vi "Find Timeout.vi"(0 "State in":refnum<class "State.lvclass">, 7 "Type":T1, 11 "error in (no error)":errorcluster) -> (4 "State thru":refnum<class "State.lvclass">, 8 "Timeout":refnum<class "Timeout.lvclass">, 15 "error out":errorcluster)   [LabVIEW 2020, in "State.lvclass"]
uses:
  State.lvclass
  Typedefs/Tosca-Event Type.ctl
  Timeout/Timeout.lvclass
  State.lvclass/State.ctl
  Timeout/Timeout.lvclass/Timeout.ctl
  Timeout/Read Type.vi
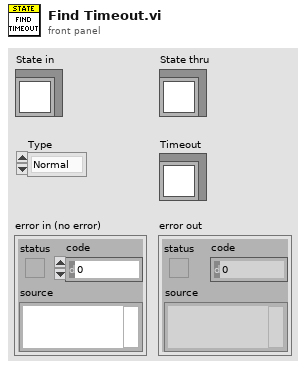
[diagram p1: front panel]
types:
  T1 = typedef "Tosca-Event Type.ctl" = enum16{"Normal", "CS+", "CS-"}
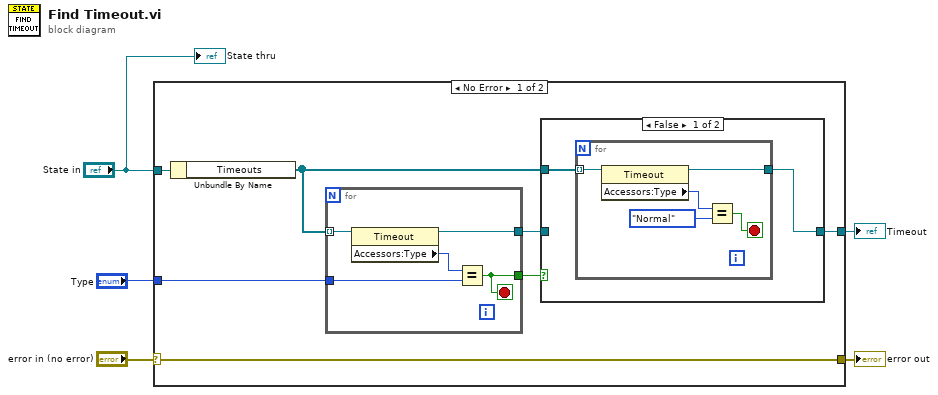
[diagram p0: block diagram]
diagram:
  n1 = case shown="No Error" "error in (no error)" {
    selector: "error in (no error)" -> [w12 w26]
    tunnel: [w12 w26] -> w4
    tunnel: "State in" -> [w11 _]
    tunnel: "Type" -> [w10 _]
    tunnel: [w8 _] -> w1
    frame No Error {
      n2 = Unbundle By Name(w11) -> ("Timeouts"=w6:refnum<class "Timeout.lvclass">[])
      n3 = for {
        tunnel: w6 -> [w17] mode=indexing
        tunnel: w10 -> [w15]
        tunnel: [w14] -> w7
        tunnel: [w13] -> w9
        stop <- w13 stop-if-true
        n4 = property class="Timeout"(reference=w17) -> (reference out=w14:refnum<class "Timeout.lvclass">, "Accessors:Type"=w16:T1)  [unwired: 1 in, 1 out]
        n5 = Equal?(x=w16, y=w15) -> (x = y?=w13:bool)
      }
      n6 = case shown="False" w9 {
        tunnel: [w18 w25] -> w8
        tunnel: w7 -> [_ w25]
        tunnel: w6 -> [w19 _]
        frame False {
          n7 = for {
            tunnel: w19 -> [w24] mode=indexing
            tunnel: [w22] -> w18
            stop <- w21 stop-if-true
            n8 = property class="Timeout"(reference=w24) -> (reference out=w22:refnum<class "Timeout.lvclass">, "Accessors:Type"=w23:T1)  [unwired: 1 in, 1 out]
            n9 = Equal?(x=w23, y=Tosca-Event_Type."Normal") -> (x = y?=w21:bool)
          }
        }
        frame True {
        }
      }
    }
    frame Error {
    }
  }
  "error out" <- w4
  "Timeout" <- w1
  "State thru" <- "State in"
